vi "Create.vi"(8 "error in (no error)":errorcluster) -> (0 "error out":errorcluster, 3 "ChartGuiTask out":refnum<class "ChartGuiTask.lvclass">)   [LabVIEW 2020, in "VolatusDemo.lvlib" / "ChartGuiTask.lvclass"]
uses:
  ChartGuiTask.lvclass
  ChartGuiTask.lvclass/ChartGuiTask.ctl
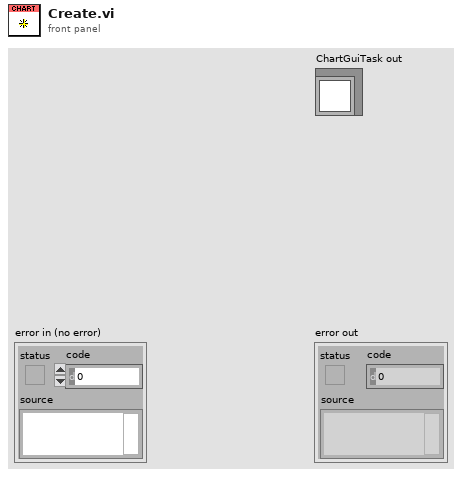
[diagram p1: front panel]
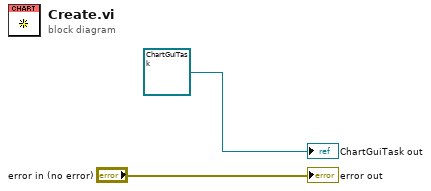
[diagram p0: block diagram]
diagram:
  "error out" <- "error in (no error)"
  "ChartGuiTask out" <- refnum<class "ChartGuiTask.lvclass"> refnum ("ChartGuiTask in")
